vi "Dim UI.vi"(8 "error in (no error)":errorcluster, 11 "Dim UI":refnum<user-event>) -> (0 "error out":errorcluster)   [LabVIEW 2020, in "Better Search.lvlib" / "BetterSearch.lvclass"]
uses:
  BetterSearch.lvclass
panel:
  # "Mouse over to return to Better Search"
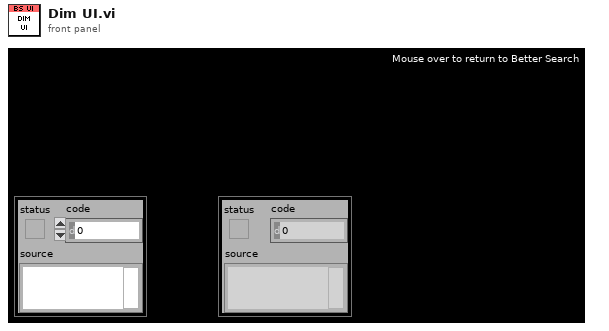
[diagram p1: front panel]
types:
  T1 = typedef "LVRectTypeDef.ctl" = cluster{"Left":i16, "Top":i16, "Right":i16, "Bottom":i16}
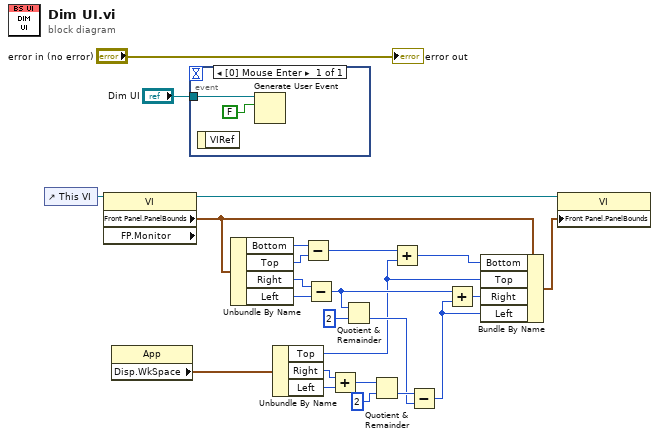
[diagram p0: block diagram]
diagram:
  n1 = control-ref of="This VI"() -> (w23:refnum<vi>)
  n2 = property class="VI" props=["Front Panel.PanelBounds", "FP.Monitor"](reference=w23) -> (reference out=w13:refnum<vi>, "Front Panel.PanelBounds"=w12:T1)  [unwired: 1 in, 2 out]
  n3 = property class="App"() -> ("Disp.WkSpace"=w7:T1)  [unwired: 2 in, 2 out]
  n4 = event shown="[0] Mouse Enter" {
    selector: _ -> [_]
    dyn-events: _ -> [_]
    timeout: _ -> [_]
    tunnel: "Dim UI" -> [w26]
    event Mouse Enter {
      n5 = event-data() -> ()  [unwired: 1 in, 1 out]
      n6 = Generate User Event(user event=w26, event data cluster=FALSE ("event data")) -> ()  [unwired: 2 in, 2 out]
    }
  }
  n7 = Unbundle By Name(w12) -> ("Bottom"=w6:i16, "Top"=w5:i16, "Right"=w16:i16, "Left"=w17:i16)
  n8 = Unbundle By Name(w7) -> ("Top"=w3:i16, "Right"=w22:i16, "Left"=w21:i16)
  n9 = Subtract(x=w6, y=w5) -> (x-y=w4:i16)
  n10 = Subtract(x=w16, y=w17) -> (x-y=w10:i16)
  n11 = Add(x=w22, y=w21) -> (x+y=w20:i16)
  n12 = Quotient & Remainder(x=w10, y=i16 2) -> (floor(x/y)=w14:i16)  [unwired: 1 out]
  n13 = Quotient & Remainder(x=w20, y=i16 2) -> (floor(x/y)=w15:i16)  [unwired: 1 out]
  n14 = Add(x=w4, y=w3) -> (x+y=w2:i16)
  n15 = Subtract(x=w15, y=w14) -> (x-y=w11:i16)
  n16 = Add(x=w10, y=w11) -> (x+y=w9:i16)
  n17 = Bundle By Name(cluster=w12, "Bottom"=w2, "Top"=w3, "Right"=w9, "Left"=w11) -> (w8:T1)
  n18 = property class="VI"(reference=w13, "Front Panel.PanelBounds"=w8) -> ()  [unwired: 1 in, 2 out]
  "error out" <- "error in (no error)"
